vi "CaseStructure.vi"() -> ()   [LabVIEW 2020]
panel:
  in  "Numeric 2":dbl
  out "Numeric":i32
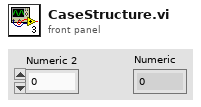
[diagram p1: front panel]
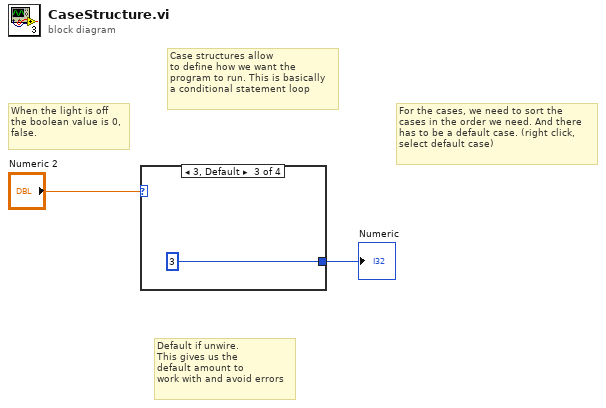
[diagram p0: block diagram]
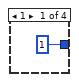
[diagram p2: hidden frame]
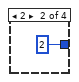
[diagram p3: hidden frame]
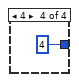
[diagram p4: hidden frame]
diagram:
  # "Default if unwire.\nThis gives us the \ndefault amount to \nwork with and avoid errors"
  # "For the cases, we need to sort the \ncases in the order we need. And there\nhas to be a default case. (right click, \nselect default case)"
  # "When the light is off\nthe boolean value is 0,\nfalse."
  # "Case structures allow\nto define how we want the\nprogram to run. This is basically\na conditional statement loop"
  n1 = case shown="3, Default" "Numeric 2" {
    tunnel: [1 2 3 4] -> w2
    frame 1 {
    }
    frame 2 {
    }
    frame 3, Default {
    }
    frame 4 {
    }
  }
  "Numeric" <- w2
